vi "SetUnits.vi"(0 "Temp":bool, 4 "SensType":i32(ring) items=["No Sensor", "Photo", "Thermo", "Pyro"], 5 "Sub1In":u16(ring)=1 caption="Sub 1" items=["Off", "Min", "Freq", "Temp", "Resistor"], 6 "Sub2In":u16(ring)=1 caption="Sub 2" items=["Off", "Max", "Ratio", "Area", "2. Unit"], 7 "MainUnitsIn":u16(ring) caption="Units" items=["W", "V", "J", "dBm", "A"]) -> (1 "Sub1Out":enum16{"Off", "Min", "Freq", "Temp", "Res"}(ring)=enum."Min", 2 "Sub2Out":u16(ring)=1 items=["Off", "Max", "Ratio", "Area", "Second"], 3 "MainUnitsOut":enum16{"W", "V", "J", "dBm", "A"}(ring))   [LabVIEW 2011]
panel:
  in  "stop":bool
  # "Set Units of Measure and\nDisplay Configuration"
  # "Power PD\n- A\n- W\n- dBm"
  # "Power TH\n- V\n- W\n- dBm"
  # "Energy\n- V\n- J"
  # "General\n- Digits"
  # "Subdisp 2\n- Maximum\n- Min/Max\n- Second Unit\n- Area"
  # "Subdisp 1\n- Temperature\n- Frequency\n- Minimum"
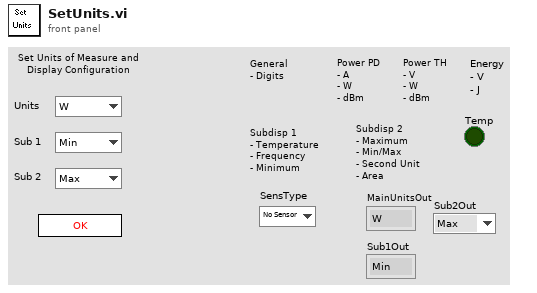
[diagram p1: front panel]
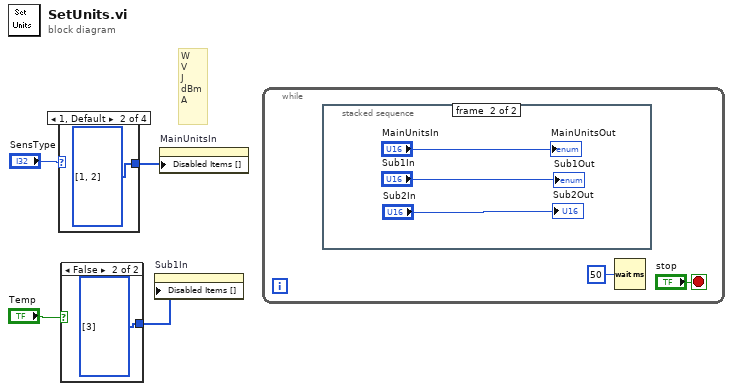
[diagram p0: block diagram]
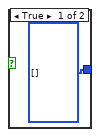
[diagram p2: hidden frame]
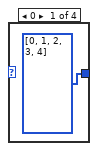
[diagram p3: hidden frame]
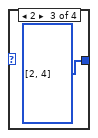
[diagram p4: hidden frame]
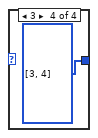
[diagram p5: hidden frame]
diagram:
  # "W\nV\nJ\ndBm\nA"
  n1 = case shown="1, Default" "SensType" {
    tunnel: [i32[] [0, 1, 2, 3, 4] ("Disabled Items []") i32[] [1, 2] ("Disabled Items []") i32[] [2, 4] ("Disabled Items []") i32[] [3, 4] ("Disabled Items []")] -> w3
    frame 0 {
    }
    frame 1, Default {
    }
    frame 2 {
    }
    frame 3 {
    }
  }
  n2 = case shown="False" "Temp" {
    tunnel: [i32[] [] ("Disabled Items []") i32[] [3] ("Disabled Items []")] -> w2
    frame True {
    }
    frame False {
    }
  }
  n3 = property on="Sub1In" class="Ring (strict)"("Disabled Items []"=w2) -> ()  [unwired: 2 in, 2 out]
  n4 = property on="MainUnitsIn" class="Ring (strict)"("Disabled Items []"=w3) -> ()  [unwired: 2 in, 2 out]
  n5 = while {
    stop <- "stop" stop-if-true
    n6 = stacked-sequence {
      frame #0 {
      }
      frame #1 {
        "MainUnitsOut" <- "MainUnitsIn"
        "Sub1Out" <- "Sub1In"
        "Sub2Out" <- "Sub2In"
      }
    }
    n7 = Wait (ms)(milliseconds to wait=u32 50) -> ()  [unwired: 1 out]
  }
